vi "Append String to Filepath.vi"(10 "Append":string, 11 "Filepath to Save Data":path) -> (3 "appended path":path)   [LabVIEW 2020]
doc: "adds the string to the file name, before the dot .file extension"
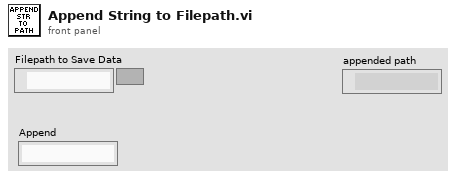
[diagram p1: front panel]
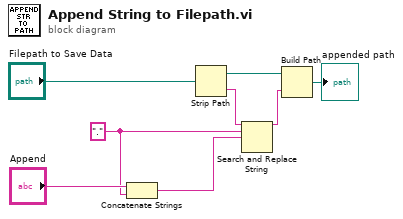
[diagram p0: block diagram]
diagram:
  w2 = "." ("search string")
  n1 = Concatenate Strings("Append", w2) -> (w1:string)
  n2 = Strip Path(path="Filepath to Save Data") -> (stripped path=w8:path, name=w6:string)
  n3 = Search and Replace String(input string=w6, search string=w2, replace string=w1) -> (result string=w7:string)  [unwired: 5 in, 3 out]
  n4 = Build Path(base path=w8, name or relative path=w7) -> (appended path=→"appended path":path)
